vi "Insert Menu Items (if not exist) Arrays.vi"(7 "menu tag":string, 8 "error in (no error)":errorcluster, 9 "Item tags":string[](array[string]), 10 "Item names":string[](array[string]), 11 "Menu in":refnum<k9>) -> (0 "error out":errorcluster, 3 "Menu out":refnum<k9>)   [LabVIEW 2019, in "Menu From Cluster.lvlib"]
uses:
  Menu From Cluster.lvlib
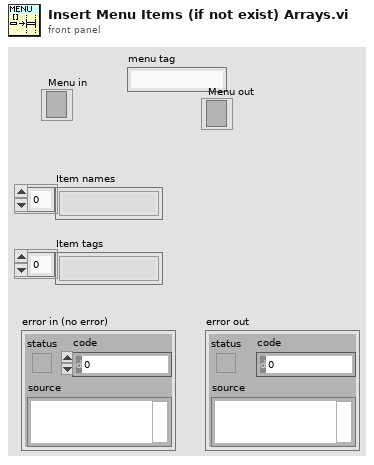
[diagram p1: front panel]
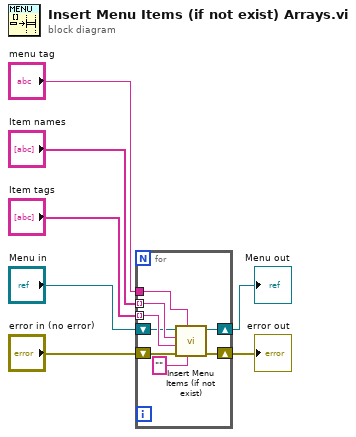
[diagram p0: block diagram]
diagram:
  n1 = for {
    tunnel: "menu tag" -> [w15]
    tunnel: "Item names" -> [w14] mode=indexing
    tunnel: "Item tags" -> [w13] mode=indexing
    shift-right: [w12] -> w4
    shift-left: "Menu in" -> [w10]
    shift-right: [w11] -> w3
    shift-left: "error in (no error)" -> [w9]
    n2 = call "Insert Menu Items (if not exist).vi"("after item"="", "menu tag"=w15, "error in (no error)"=w9, "item tag"=w13, "item name"=w14, "Menu in"=w10) -> ("error out"=w11:errorcluster, "Menu out"=w12:refnum<k9>)  [unwired: 3 in, 1 out]
  }
  "Menu out" <- w4
  "error out" <- w3
